vi "GetType.vi"(8 "error in (no error)":errorcluster, 11 "Configure Trigger Source [TRG] Msg":refnum<class "Configure Trigger Source [TRG] Msg.lvclass">) -> (0 "error out":errorcluster, 2 "Data Sample":variant, 3 "Configure Trigger Source [TRG] Msg":refnum<class "Configure Trigger Source [TRG] Msg.lvclass">)   [LabVIEW 2015, in "CS++Fgen.lvlib" / "Configure Trigger Source [TRG] Msg.lvclass"]
doc: "This VI delivers a sample of the data type format the message expects."
uses:
  Configure Trigger Source [TRG] Msg.lvclass
  Configure Trigger Source [TRG] Msg.lvclass/Configure Trigger Source [TRG] Msg.ctl
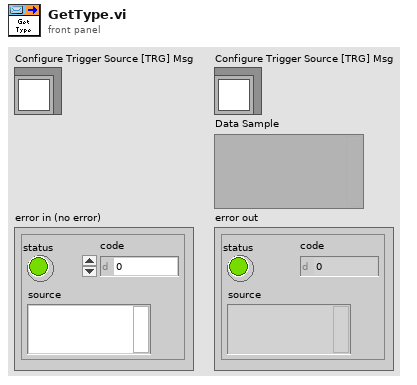
[diagram p1: front panel]
types:
  T1 = cluster{"channel name (\"CHANNEL1\")":string, "trigger source (External)":i32}
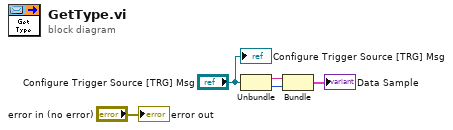
[diagram p0: block diagram]
diagram:
  n1 = Unbundle("Configure Trigger Source [TRG] Msg") -> (w2:string, w1:i32)
  n2 = Bundle("channel name (\"CHANNEL1\")"=w2, "trigger source (External)"=w1) -> (→"Data Sample":T1)  [unwired: 1 in]
  "error out" <- "error in (no error)"
  "Configure Trigger Source [TRG] Msg" <- "Configure Trigger Source [TRG] Msg"
